vi "Stop Output.vi"(8 "error in (no error)":errorcluster, 11 "Hardware Configuration In":T1={"Task ID"=0, "Volume"=0.0, "Data"={"SignalType"=enum."SineWave", "WhiteNoiseSettings"={"Generate New Data"=FALSE, "Save"=FALSE, "Filter"=TRUE, "Gain"=0}, "SineWaveSttings"={"Frequency"=0.0, "Amplitude"=0.0}}, "Generated Data"={"t0"=timestamp(0 s since 1904-01-01), "dt"=1.0, "Y"=[]}} {"task ID out" format="%.0x"}) -> (0 "error out":errorcluster)   [LabVIEW 2022 SP3]
doc: "Stops the acquisition."
uses:
  Output Hardware Configuration.ctl
  <vilib>/sound2/lvsound2.llb/Sound Output Task ID.ctl
  Data.ctl
  WhiteNoiseSettings.ctl
  SineWaveSettings.ctl
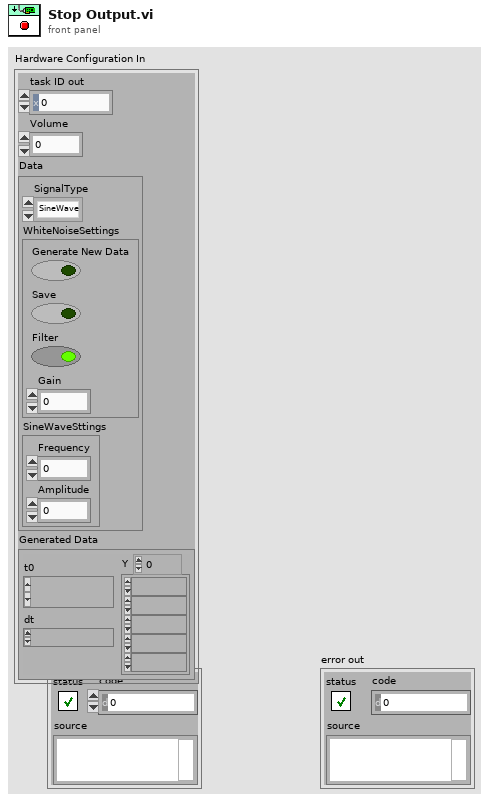
[diagram p1: front panel]
types:
  T1 = typedef "Output Hardware Configuration.ctl" = cluster{"Task ID":T2, "Volume":dbl, "Data":T3, "Generated Data":waveform(dbl)}
  T2 = typedef "Sound Output Task ID.ctl" = u32
  T3 = typedef "Data.ctl" = cluster{"SignalType":enum16{"WhiteNoise", "SineWave"}, "WhiteNoiseSettings":T4, "SineWaveSttings":T5}
  T4 = typedef "WhiteNoiseSettings.ctl" = cluster{"Generate New Data":bool, "Save":bool, "Filter":bool, "Gain":i32}
  T5 = typedef "SineWaveSettings.ctl" = cluster{"Frequency":dbl, "Amplitude":dbl}
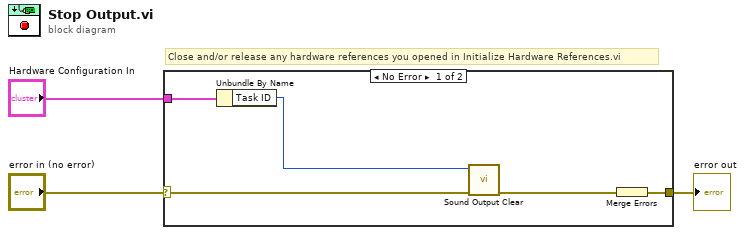
[diagram p0: block diagram]
diagram:
  # "Close and/or release any hardware references you opened in Initialize Hardware References.vi"
  n1 = case shown="No Error" "error in (no error)" {
    selector: "error in (no error)" -> [w6 w9]
    tunnel: [w8 w9] -> w2
    tunnel: "Hardware Configuration In" -> [w7 _]
    frame No Error {
      n2 = Unbundle By Name(w7) -> ("Task ID"=w5:T2)
      n3 = call <vilib>:"Sound Output Clear.vi"("error in (no error)"=w6, "task ID"=w5) -> ("error out"=w4:errorcluster)  [unwired: 9 in]
      n4 = Merge Errors(w4) -> (w8:errorcluster)
    }
    frame Error {
    }
  }
  "error out" <- w2
